vi "get_config_cluster.vi"(8 "error in (no error)":errorcluster, 11 "ScanHeadDL090202 in":refnum<class "ScanHeadDL090202.lvclass">) -> (0 "error out":errorcluster, 2 "config cluster (variant)":variant, 3 "ScanHeadDL090202 out":refnum<class "ScanHeadDL090202.lvclass">)   [LabVIEW 2010, in "ScanHeadDL090202.lvclass"]
uses:
  ScanHeadDL090202.lvclass
  ScanHeadDL090202.lvclass/ScanHeadDL090202.ctl
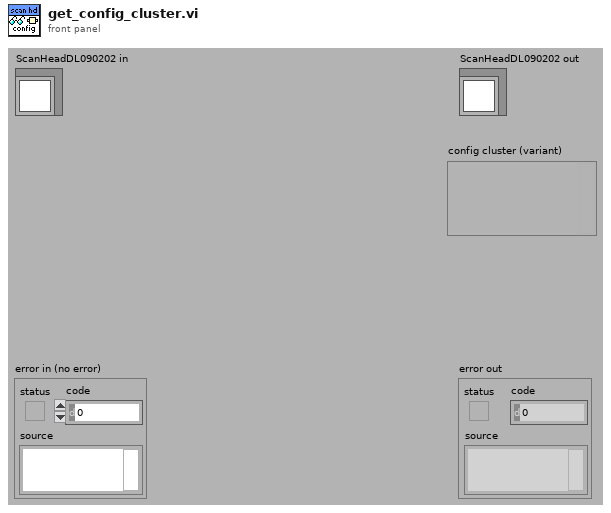
[diagram p1: front panel]
types:
  T1 = typedef "ScanHeadDL090202.lvclass/config_data_cluster.ctl" = cluster{"subcomponents":T2, "scanner factors":dbl[unit][], "modifier factor":dbl, "LSID":T4, "visibility":cluster{"Zoom":bool, "RotateX":bool, "RotateZ":bool, "TranslateX":bool, "TranslateY":bool, "TranslateZ":bool}, "available settings":T5[], "default settings":string}
  T2 = typedef "ScanHeadDL090202.lvclass/subcomponent_specifications_cluster.ctl" = cluster{"scanners":T3[], "intensity modifier":T3, "clock":T3, "shutter":T3}
  T3 = typedef "plugin_specification.ctl" = cluster{"class path":string, "configuration":string, "label":string, "settings name":string}
  T4 = typedef "LSID_cluster.ctl" = cluster{"identifier":string, "revision":i32}
  T5 = typedef "settings_specification_cluster.ctl" = cluster{"name":string, "label":string}
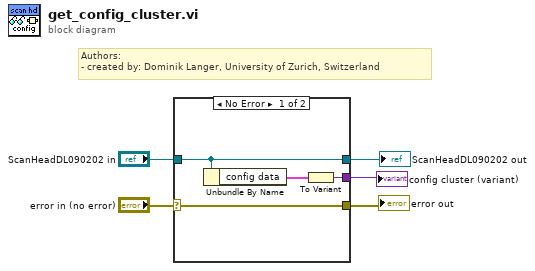
[diagram p0: block diagram]
diagram:
  # "Authors: \n- created by: Dominik Langer, University of Zurich, Switzerland"
  n1 = case shown="No Error" "error in (no error)" {
    selector: "error in (no error)" -> [w6 w11]
    tunnel: "ScanHeadDL090202 in" -> [w9 w10]
    tunnel: [w7 _] -> w1
    tunnel: [w6 w11] -> w3
    tunnel: [w9 w10] -> w2
    frame No Error {
      n2 = Unbundle By Name(w9) -> ("config data"=w8:T1)
      n3 = To Variant(anything=w8) -> (Variant=w7:variant)
    }
    frame Error {
    }
  }
  "error out" <- w3
  "ScanHeadDL090202 out" <- w2
  "config cluster (variant)" <- w1
